vi "Apply Firmware.vi"(7 "Installation Notifiers":T1, 8 "error in":errorcluster caption="error in (no error)", 11 "Target settings":T2={"Hostname"="", "Serial number"="", "Product name"="", "Product code"=0, "System status"="", "Credential type"=enum."None/Unlocked", "User added?"=FALSE, "Primary NIC"={"MAC address"="", "IP Address Request Mode"=2, "IP address"="", "Subnet mask"="", "Gateway"="", "DNS server"=""}, "System Credentials"={"Username"="", "Password"=""}} {"Primary NIC"."IP Address Request Mode" items=["Static"=1, "DHCP/Link-Local"=2, "Link-Local Only"=4, "DHCP Only"=8]}) -> (0 "error out":errorcluster, 2 "Detailed Result":string, 3 "Firmware Status":T5=2 items=["update pending auto restart"=-4, "verifying new image"=-3, "writing/flashing new image"=-2, "waiting for image"=-1, "corrupt firmware, cannot run"=0, "no firmware installed"=1, ""=2, "update pending user restart"=3, "update pending user action"=4, "update attempt failed"=5])   [LabVIEW 2020]
doc: "This Vi will upgrade the RT device's firmware if it is not supported by SystemLink Client, which means firmware must be higher than version 6."
uses:
  <vilib>/nisyscfg/Firmware Status.ctl
  Controls/Target Information.ctl
  Controls/Target Network Settings.ctl
  Controls/System Credentials.ctl
  Controls/Installation Notifiers.ctl
  Controls/Deployment Status Data Type.ctl
  Controls/Deployment Progress Data Type.ctl
  <vilib>/nisyscfg/Upgrade Firmware (File).vi
  <vilib>/nisyscfg/Close (Hardware).vi
  <vilib>/nisyscfg/Close (System).vi
  <resource>/objmgr/nisysapi.rc
  <vilib>/nisyscfg/nisyscfg.lvlib
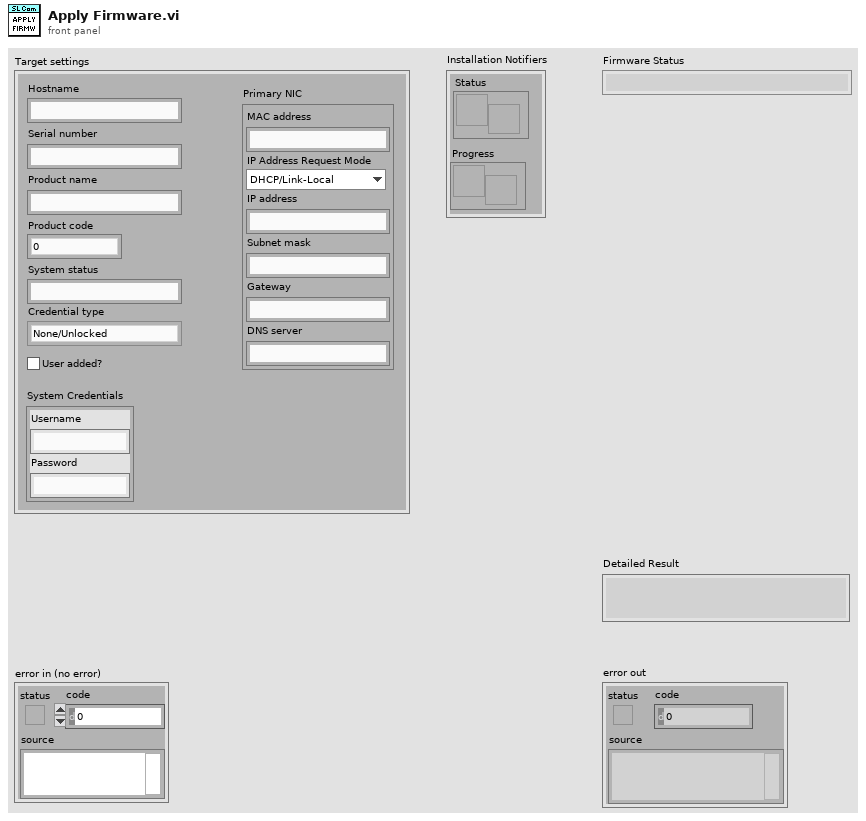
[diagram p1: front panel]
types:
  T1 = typedef "Installation Notifiers.ctl" = cluster{"Status":refnum<notifier>, "Progress":refnum<notifier>}
  T2 = typedef "Target Information.ctl" = cluster{"Hostname":string, "Serial number":string, "Product name":string, "Product code":i32, "System status":string, "Credential type":enum16{"None/Unlocked", "FTP Password", "NIAuth Credentials"}, "User added?":bool, "Primary NIC":T3, "System Credentials":T4}
  T3 = typedef "Target Network Settings.ctl" = cluster{"MAC address":string, "IP Address Request Mode":i32, "IP address":string, "Subnet mask":string, "Gateway":string, "DNS server":string}
  T4 = typedef "System Credentials.ctl" = cluster{"Username":string, "Password":string}
  T5 = typedef "nisyscfg.lvlib/Firmware Status.ctl" = i32
  T6 = typedef "Deployment Status Data Type.ctl" = string
  T7 = typedef "Deployment Progress Data Type.ctl" = i8
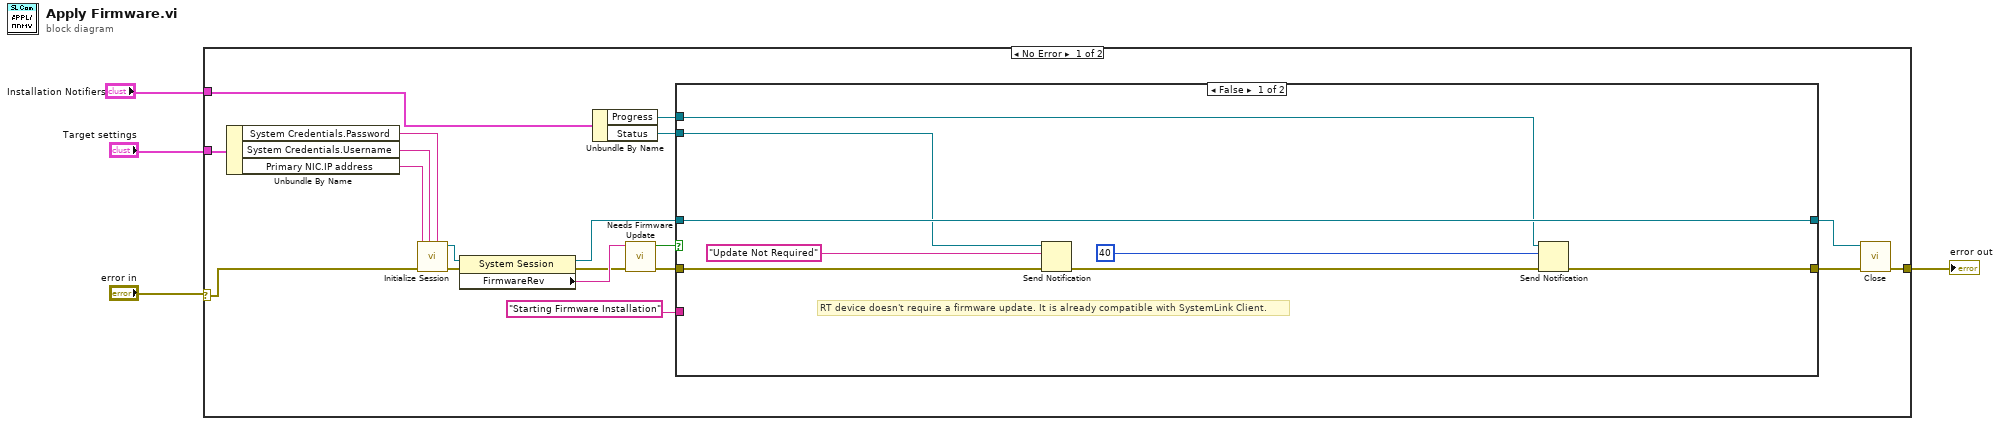
[diagram p0: block diagram]
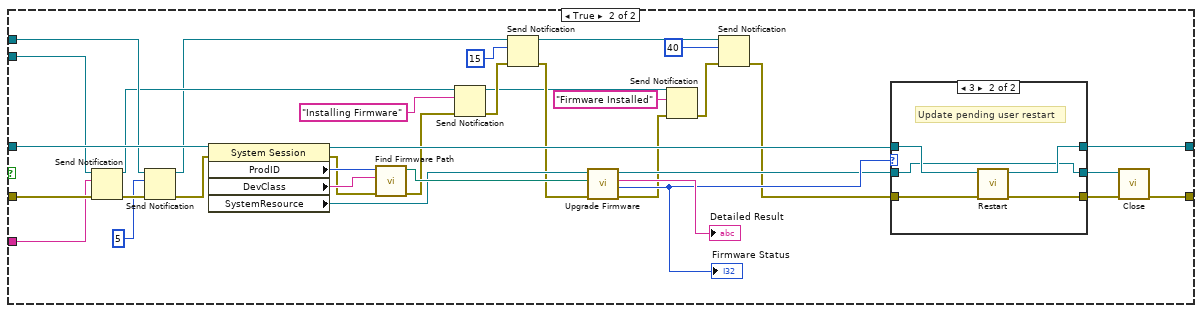
[diagram p2: hidden frame]
diagram:
  n1 = case shown="No Error" "error in" {
    selector: "error in" -> [w14 w75]
    tunnel: [w23 w75] -> w2
    tunnel: "Target settings" -> [w20 _]
    tunnel: "Installation Notifiers" -> [w8 _]
    frame No Error {
      n2 = Unbundle By Name(w20) -> ("System Credentials.Password"=w9:string, "System Credentials.Username"=w10:string, "Primary NIC.IP address"=w19:string)
      n3 = call <vilib>:"Initialize Session.vi"("Password"=w9, "User Name"=w10, "error in (no error)"=w14, "Target (localhost)"=w19) -> ("error out"=w22:errorcluster, "Session out"=w21:refnum<k21>)  [unwired: 6 in]
      n4 = property class="System Session"(reference=w21, error in=w22) -> (reference out=w16:refnum<k21>, error out=w17:errorcluster, "FirmwareRev"=w18:string)
      n5 = Unbundle By Name(w8) -> ("Progress"=w7:refnum<notifier>, "Status"=w6:refnum<notifier>)
      n6 = call "Needs Firmware Update.vi"("error in (no error)"=w17, "FirmwareRev"=w18) -> ("error out"=w12:errorcluster, "Update?"=w13:bool)  [unwired: 8 in]
      n7 = case shown="False" w13 {
        tunnel: w12 -> [w30 w52]
        tunnel: w16 -> [w31 w62]
        tunnel: [w31 w64] -> w15
        tunnel: [w28 w55] -> w11
        tunnel: w7 -> [w25 w45]
        tunnel: w6 -> [w24 w46]
        tunnel: T6 "Starting Firmware Installation" ("notification") -> [_ w49]
        frame False {
          # "RT device doesn't require a firmware update. It is already compatible with SystemLink Client."
          n8 = Send Notification(notification=T6 "Update Not Required", notifier=w24, error in (no error)=w30) -> (error out=w29:errorcluster)  [unwired: 1 out]
          n9 = Send Notification(notification=T7 40, notifier=w25, error in (no error)=w29) -> (error out=w28:errorcluster)  [unwired: 1 out]
        }
        frame True {
          n10 = Send Notification(notification=w49, notifier=w46, error in (no error)=w52) -> (notifier out=w35:refnum<notifier>, error out=w51:errorcluster)
          n11 = Send Notification(notification=T7 5, notifier=w45, error in (no error)=w51) -> (notifier out=w34:refnum<notifier>, error out=w50:errorcluster)
          n12 = property class="System Session"(reference=w62, error in=w50) -> (reference out=w57:refnum<k21>, error out=w59:errorcluster, "ProdID"=w61:i32, "DevClass"=w60:string, "SystemResource"=w53:refnum<k20>)
          n13 = call "Find Firmware Path.vi"("error in"=w59, "Device Class"=w60, "Product ID"=w61) -> ("error out"=w44:errorcluster, "Firmware Path"=w58:path)  [unwired: 7 in]
          n14 = Send Notification(notification=T6 "Installing Firmware", notifier=w35, error in (no error)=w44) -> (notifier out=w36:refnum<notifier>, error out=w47:errorcluster)
          n15 = Send Notification(notification=T7 15, notifier=w34, error in (no error)=w47) -> (notifier out=w37:refnum<notifier>, error out=w43:errorcluster)
          n16 = call-poly <vilib>:"Upgrade Firmware.vi"("error in (no error)"=w43, "Firmware File"=w58, "Resource in"=w53) -> ("error out"=w40:errorcluster, "Firmware Status"=w65:T5, "Detailed Result"=→"Detailed Result":string, "Resource out"=w63:refnum<k20>)  [unwired: 5 in]
          "Firmware Status" <- w65
          n17 = Send Notification(notification=T6 "Firmware Installed", notifier=w36, error in (no error)=w40) -> (error out=w38:errorcluster)  [unwired: 1 out]
          n18 = Send Notification(notification=T7 40, notifier=w37, error in (no error)=w38) -> (error out=w39:errorcluster)  [unwired: 1 out]
          n19 = case shown="3" w65 {
            tunnel: w39 -> [w68 w74]
            tunnel: w57 -> [w69 w73]
            tunnel: [w69 w72] -> w64
            tunnel: [w68 w71] -> w56
            tunnel: w63 -> [w67 w70]
            tunnel: [w67 w70] -> w54
            frame 0, Default {
            }
            frame 3 {
              # "Update pending user restart"
              n20 = call <vilib>:"Restart.vi"("error in (no error)"=w74, "Session in"=w73) -> ("error out"=w71:errorcluster, "Session out"=w72:refnum<k21>)  [unwired: 7 in, 1 out]
            }
          }
          n21 = call-poly <vilib>:"Close.vi"("error in (no error)"=w56, "Resource in"=w54) -> ("error out"=w55:errorcluster)  [unwired: 9 in]
        }
      }
      n22 = call-poly <vilib>:"Close.vi"("error in (no error)"=w11, "Session in"=w15) -> ("error out"=w23:errorcluster)  [unwired: 9 in]
    }
    frame Error {
    }
  }
  "error out" <- w2
